vi "国标仪器启动命令.vi"(8 "error in (no error)":errorcluster, 11 "参数":T1={"站号"=1, "量程切换"=enum."AUTO", "控制命令"=enum."启动测量", "模式设置"=enum."待机", "测量间隔"=0} {"站号" items=["总磷"=1, "总氮"=2, "氨氮"=3, "CODMn"=21]}) -> (0 "error out":errorcluster)   [LabVIEW 2016, in "质控单元V1.lvlib"]
uses:
  <vilib>/Plasmionique/MB Master/MB_Master/MB_Master.lvclass
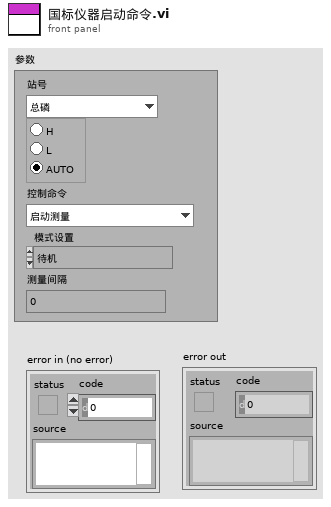
[diagram p1: front panel]
types:
  T1 = cluster{"站号":u16, "量程切换":enum32{"H", "L", "AUTO"}, "控制命令":enum16{"启动测量", "标样核查", "零点核查", "跨度核查", "空白测试", "平行样测试", "加标回收", "空白校准", "标样校准", "初始化（清洗）", "停止测试", "仪器重启", "校时", "模式设置", "测量间隔设置"}, "模式设置":enum16{"待机", "连续模式", "周期模式", "定点模式", "受控模式", "手动模式"}, "测量间隔":u16}
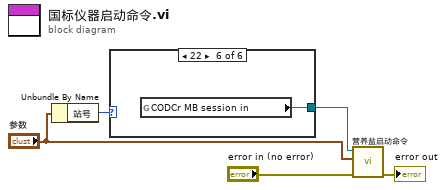
[diagram p0: block diagram]
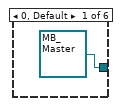
[diagram p2: hidden frame]
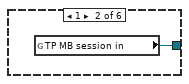
[diagram p3: hidden frame]
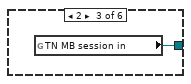
[diagram p4: hidden frame]
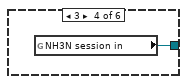
[diagram p5: hidden frame]
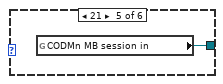
[diagram p6: hidden frame]
diagram:
  n1 = Unbundle By Name("参数") -> ("站号"=w3:u16)
  n2 = case shown="22" w3 {
    tunnel: [refnum<class "MB_Master.lvclass"> refnum ("CODMn MB session in") w7 w8 w9 w10 w11] -> w5
    frame 0, Default {
    }
    frame 1 {
      n3 = global read "系统交互.vi" "TP MB session in"() -> (w7:refnum<class "MB_Master.lvclass">)
    }
    frame 2 {
      n4 = global read "系统交互.vi" "TN MB session in"() -> (w8:refnum<class "MB_Master.lvclass">)
    }
    frame 3 {
      n5 = global read "系统交互.vi" "NH3N session in"() -> (w9:refnum<class "MB_Master.lvclass">)
    }
    frame 21 {
      n6 = global read "系统交互.vi" "CODMn MB session in"() -> (w10:refnum<class "MB_Master.lvclass">)
    }
    frame 22 {
      n7 = global read "系统交互.vi" "CODCr MB session in"() -> (w11:refnum<class "MB_Master.lvclass">)
    }
  }
  n8 = call "营养盐启动命令.vi"("error in (no error)"="error in (no error)", "参数"="参数", "MB session in"=w5) -> ("error out"=→"error out":errorcluster)  [unwired: 8 in]
